vi "FireStatusEvent.vi"(0 "object in":refnum<class "Application.lvclass">, 2 "Status":string, 5 "error in (no error)":errorcluster) -> (14 "object out":refnum<class "Application.lvclass">, 19 "error out":errorcluster)   [LabVIEW 2019, in "Application.lvclass"]
uses:
  Application.lvclass
  Application.lvclass/Application.ctl
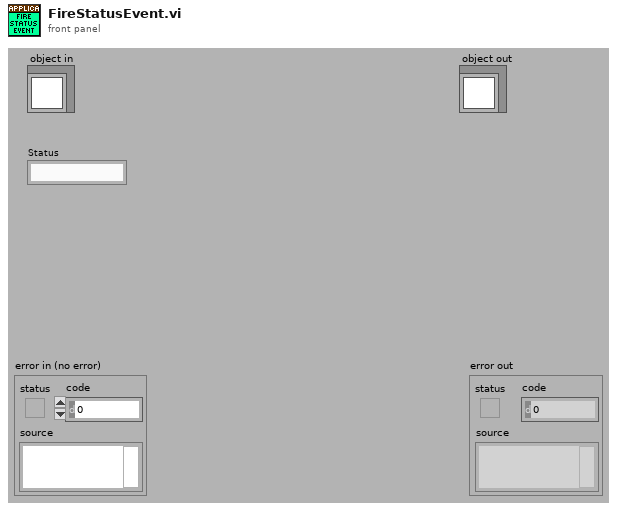
[diagram p1: front panel]
types:
  T1 = cluster{"Message":string, "Message Data":variant}
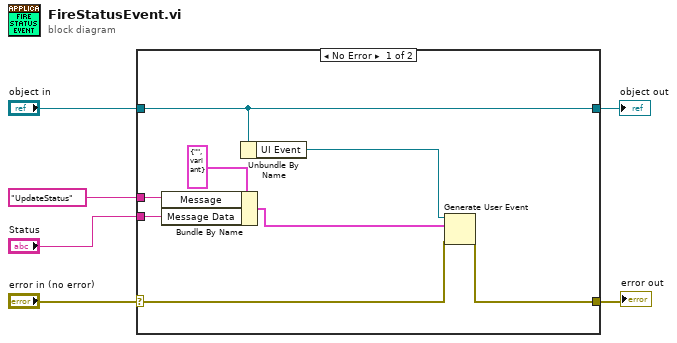
[diagram p0: block diagram]
diagram:
  n1 = case shown="No Error" "error in (no error)" {
    selector: "error in (no error)" -> [w12 w16]
    tunnel: [w11 w16] -> w5
    tunnel: [w14 w15] -> w3
    tunnel: "object in" -> [w14 w15]
    tunnel: "UpdateStatus" ("UpdateStatus") -> [w8 _]
    tunnel: "Status" -> [w7 _]
    frame No Error {
      n2 = Bundle By Name(cluster=T1 {"Message"="", "Message Data"=variant} ("event data"), "Message"=w8, "Message Data"=w7) -> (w9:T1)
      n3 = Unbundle By Name(w14) -> ("UI Event"=w13:refnum<user-event>)
      n4 = Generate User Event(user event=w13, event data cluster=w9, error in=w12) -> (error out=w11:errorcluster)  [unwired: 1 in, 1 out]
    }
    frame Error {
    }
  }
  "error out" <- w5
  "object out" <- w3
